vi "ViewProject.vi"() -> ()   [LabVIEW 2020]
uses:
  <vilib>/Instr/_visa.llb/VISA Configure Serial Port (Instr).vi
panel:
  out "CM":dbl(slide) scale=0.0..15.0
  out "CHART":dbl(graph)
  out "DISTANCE (CM)":dbl caption="Numeric" format="%_2f"
  out "read buffer":string
  out "error out":errorcluster
  in  "stop":bool
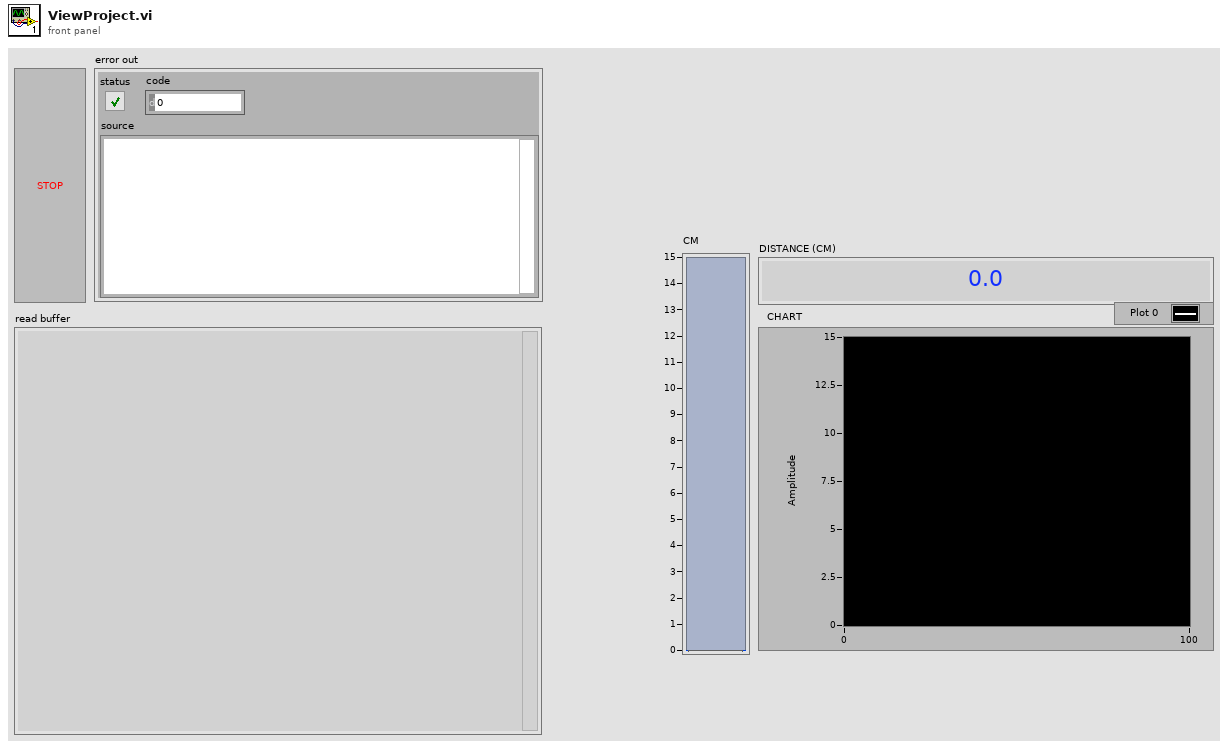
[diagram p1: front panel]
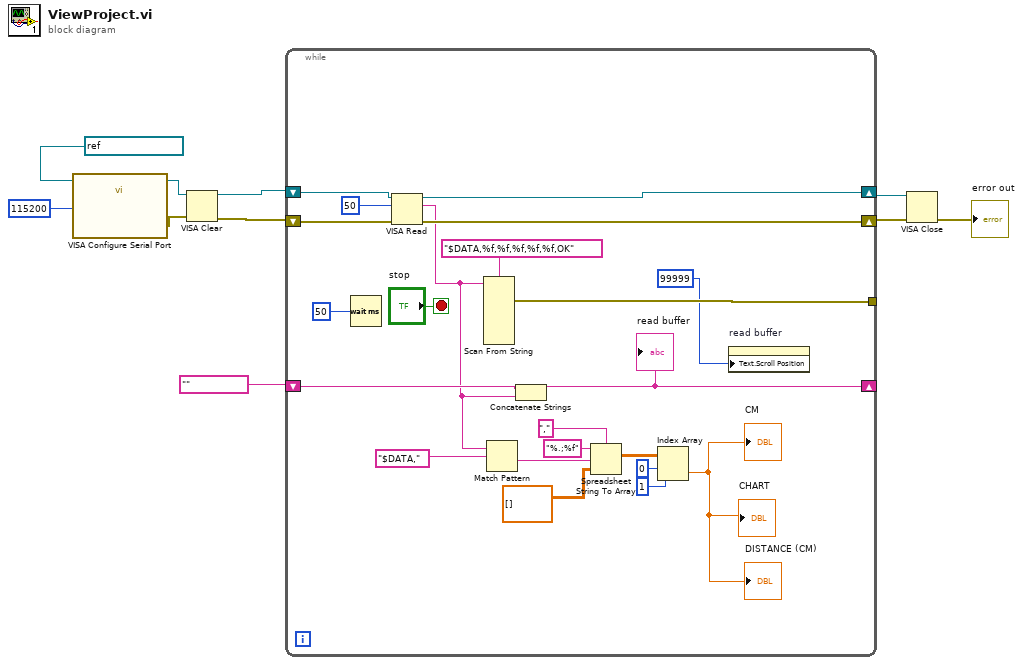
[diagram p0: block diagram]
diagram:
  n1 = call-poly "VISA Configure Serial Port"("VISA resource name"=refnum<visa-resource-name> "ASRL3::INSTR", "baud rate (9600)"=u32 115200) -> ("VISA resource name out"=w3:refnum<visa-resource-name>, "error out"=w2:errorcluster)  [unwired: 12 in]
  n2 = VISA Clear(VISA resource name=w3, error in (no error)=w2) -> (VISA resource name out=w4:refnum<visa-resource-name>, error out=w1:errorcluster)
  n3 = while {
    shift-right: [w32] -> w9
    shift-left: w4 -> [w14]
    shift-right: [w28] -> w10
    shift-left: w1 -> [w13]
    tunnel: [w27] -> _
    shift-right: [w25] -> _
    shift-left: "" -> [w26]
    stop <- "stop" stop-if-true
    n4 = Wait (ms)(milliseconds to wait=u32 50) -> ()  [unwired: 1 out]
    n5 = VISA Read(VISA resource name=w14, byte count=u32 50, error in (no error)=w13) -> (VISA resource name out=w32:refnum<visa-resource-name>, read buffer=w24:string, error out=w28:errorcluster)  [unwired: 1 out]
    n6 = Scan From String(format string="$DATA,%f,%f,%f,%f,%f,OK", input string=w24) -> (error out=w27:errorcluster)  [unwired: 12 in, 2 out]
    n7 = Match Pattern(string=w24, regular expression="$DATA," ("format string")) -> (after substring=w22:string)  [unwired: 1 in, 3 out]
    n8 = Concatenate Strings(w26, w24) -> (w25:string)
    "read buffer" <- w25
    n9 = Spreadsheet String To Array(delimiter (Tab)="," ("format string"), format string="%.;%f", spreadsheet string=w22, array type (2D Dbl)=dbl[][] []) -> (array=w21:dbl[][])
    n10 = Index Array(array=w21, index (row)=0, index (col)=1 ("disabled index (col)")) -> (element=→"CHART" →"DISTANCE (CM)" →"CM":dbl)
    n11 = property on="read buffer" class="Str"("Text.Scroll Position"=u32 99999) -> ()  [unwired: 2 in, 2 out]
  }
  n12 = VISA Close(VISA resource name=w9, error in (no error)=w10) -> (error out=→"error out":errorcluster)
